vi "Case Structure - Selector Data Types.vi"() -> ()   [LabVIEW 2023]
doc: "Illustrates the different data types that can be wired to the Case Selector terminal of a Case Structure. A Case Selector terminal can accept one of five possible data types: Boolean, error cluster, integer, enum, or string."
uses:
  support/Case Structure - Enum Options.ctl
panel:
  in  "String":string
  in  "Enum":T1
  in  "Integer":i32
  in  "Error":errorcluster
  in  "Boolean":bool
  # "Overview: Illustrates the different data types that can be wired to the Case Selector terminal of a Case Structure.\nInstructions:\nOpen the block diagram of this VI to see all the possible data types that can be wired to the Case Selector terminal of a Case Structure."
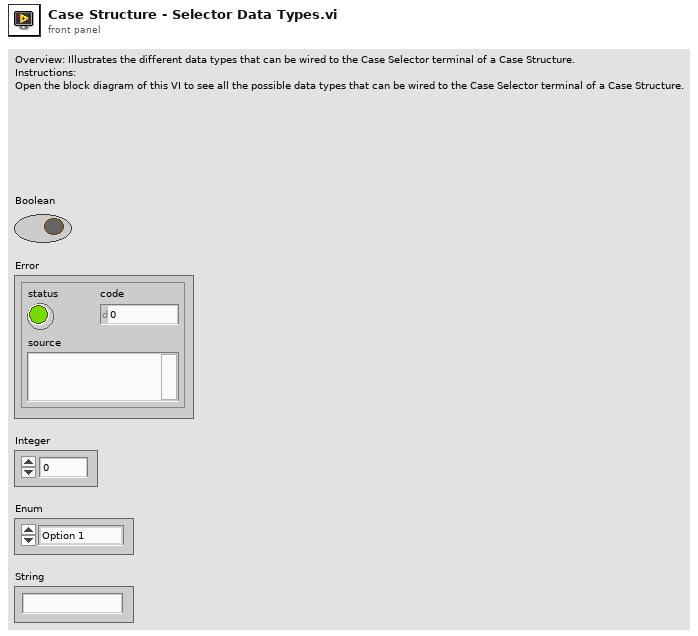
[diagram p1: front panel]
types:
  T1 = typedef "Case Structure - Enum Options.ctl" = enum16{"Option 1", "Option 2", "Option 3", "Option 4", "Option 5"}
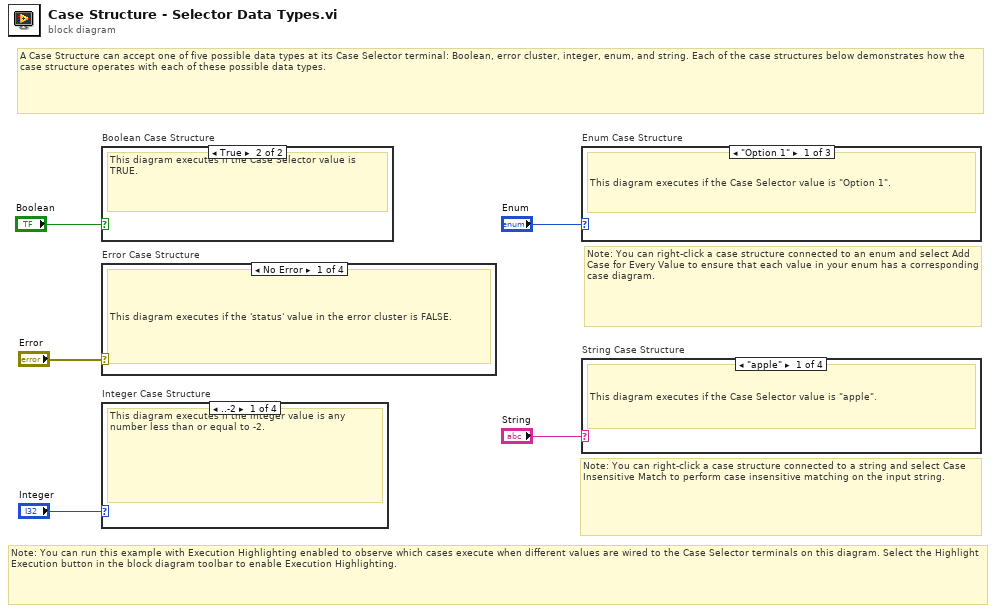
[diagram p0: block diagram]
diagram:
  # "Note: You can right-click a case structure connected to a string and select Case Insensitive Match to perform case insensitive matching on the input string."
  # "Note: You can right-click a case structure connected to an enum and select Add Case for Every Value to ensure that each value in your enum has a corresponding case diagram."
  # "A Case Structure can accept one of five possible data types at its Case Selector terminal: Boolean, error cluster, integer, enum, and string. Each of the case structures below demonstrates how the case structure operates with each of these possible data types."
  # "Note: You can run this example with Execution Highlighting enabled to observe which cases execute when different values are wired to the Case Selector terminals on this diagram. Select the Highlight Execution button in the block diagram toolbar to enable Execution Highlighting."
  n1 = case "Boolean Case Structure" shown="True" "Boolean" {
    frame False {
      # "This diagram executes if the Case Selector value is FALSE."
    }
    frame True {
      # "This diagram executes if the Case Selector value is TRUE."
    }
  }
  n2 = case "Error Case Structure" shown="No Error" "Error" {
    frame No Error {
      # "This diagram executes if the 'status' value in the error cluster is FALSE."
    }
    frame Error {
      # "This diagram executes if the 'status' value in the error cluster is TRUE and the 'code' value in the error cluster is any value between 1 and 5. Note: Specify a range of \"Error ..\" to handle all error code values."
    }
    frame Error {
      # "This diagram executes if the 'status' value in the error cluster is TRUE and the 'code' value in the error cluster is 6, 10, or 20."
    }
    frame Default {
      # "This diagram executes if the 'status' value in the error cluster is TRUE and the 'code' value in the error cluster is any value other than the values and ranges defined in the other 'Error' cases."
    }
  }
  n3 = case "Integer Case Structure" shown="..-2" "Integer" {
    frame ..-2 {
      # "This diagram executes if the integer value is any number less than or equal to -2."
    }
    frame -1, 1, 3 {
      # "This diagram executes if the integer value is -1, 1, or 3."
    }
    frame 0, 2, 4..9 {
      # "This diagram executes if the integer value is 0, 2, or any number between 4 and 9 (inclusive)."
    }
    frame Default {
      # "This diagram executes if the integer value is anything other than what is specified in the other cases of this case structure."
    }
  }
  n4 = case "Enum Case Structure" shown="\"Option 1\"" "Enum" {
    frame "Option 1" {
      # "This diagram executes if the Case Selector value is \"Option 1\"."
    }
    frame "Option 2".."Option 4" {
      # "This diagram executes if the Case Selector value is \"Option 2\", \"Option 3\", or \"Option 4\"."
    }
    frame Default {
      # "This diagram executes if the enum value is anything other than what is specified in the other cases of this case structure."
    }
  }
  n5 = case "String Case Structure" shown="\"apple\"" "String" {
    frame "apple" {
      # "This diagram executes if the Case Selector value is \"apple\"."
    }
    frame "lemon", "orange" {
      # "This diagram executes if the Case Selector value is \"lemon\" or \"orange\"."
    }
    frame "" {
      # "This diagram executes if the Case Selector value is an empty string."
    }
    frame Default {
      # "This diagram executes if the string value is anything other than what is specified in the other cases of this case structure."
    }
  }
